vi "gyro-sweeper-module-V3.vi"(8 "fitter event pair":T4, 9 "async sweeper event pair":T4, 11 "this sweeper event pair":T4) -> ()   [LabVIEW 2018]
uses:
  cursor winow.ctl
  cursor window action.ctl
  KM_file -- read-write control.ctl
  filename-action.ctl
  file -- read-write control.ctl
  publisher action.ctl
  show-win- control.ctl
  server talkto message type.ctl
  filename-pattern.ctl
  server talkback message type.ctl
  server talk-to-back pair.ctl
panel:
  in  "sweeper panel":T1(tab)
  in  "sweep is ON":bool
  in  "win":T2={"cen (Hz)"=70746.20478327299, "win (Hz)"=2974.673840305428, "left (Hz)"=69258.86786312028, "right (Hz)"=72233.5417034257}
  out "Plot: circle sweep window":cluster{"Freq out (Hz)":dbl[], dbl[]}[](graph)
  in  "sweep! :r":bool
  in  "subtract bgnd!":bool
  in  "fit!":bool=TRUE
  in  "cursor window":T3={"left"=69258.86786312028, "right "=72233.5417034257, "center"=70746.20478327299, "window"=2974.673840305428, "cursors"=[0, 1, 2], "relative"=0, "absolute"=0, "fixed vertical offset"=0.0, "vertical offset"=0.0, "skew"=0.0, "default window frac"=0.1, "kind"=enum."symmetric", "skew.left"=0.5, "skew.right"=0.5, "Plot ref"=refnum, "wing order"=enum."forw"}
  in  "save data":enum32{"save/read"}(tab)
  in  "freqsweep name template":T5={"prefix"="RuCl3-rod", "group"="f"}
  in  "Save folder":path=path "/Users/Shared/Data"
  in  "freq sweep file name":string="f020_RuCl3-rod_042518.dat"
  in  "read from disk :l":bool
  in  "read file":path=path "/Users/arkady/Desktop/local_data/TaAs-quirk-Jan2018-losalamos/9w/f006_rucl3_012518.dat"
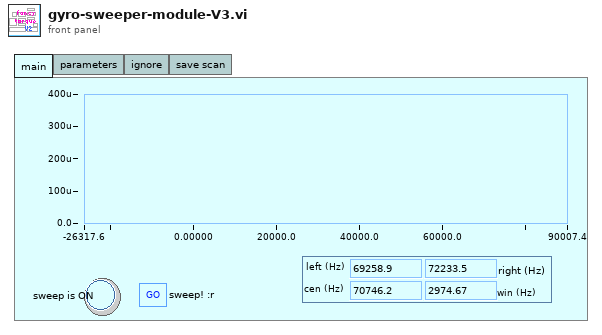
[diagram p1: front panel]
types:
  T1 = enum32{"main", "parameters", "ignore", "save scan"}
  T2 = typedef "show-win- control.ctl" = cluster{"cen (Hz)":dbl, "win (Hz)":dbl, "left (Hz)":dbl, "right (Hz)":dbl}
  T3 = typedef "cursor winow.ctl" = cluster{"left":dbl, "right ":dbl, "center":dbl, "window":dbl, "cursors":i32[], "relative":i32, "absolute":i32, "fixed vertical offset":dbl, "vertical offset":dbl, "skew":dbl, "default window frac":dbl, "kind":enum16{"symmetric", "skewed", "fancy"}, "skew.left":dbl, "skew.right":dbl, "Plot ref":refnum<vi>, "wing order":enum16{"forw", "back"}}
  T4 = typedef "server talk-to-back pair.ctl" = cluster{"talkback event":refnum<user-event>, "talkto event":refnum<user-event>}
  T5 = typedef "filename-pattern.ctl" = cluster{"prefix":string, "group":string}
  T6 = typedef "cursor window action.ctl" = enum16{"balance", "h. offset change", "cursor moves", "change center", "change window", "init", "check", "reset", "set y to middle", "idle", "-write all Y", "-write left.X", "-write center.X", "-write right.X", "-write all X", "-change center", "-change window", "-change skew", "-read cursor 2", "-read cursor 1", "-read cursor 0", "-read all cursors", "-reset", "-read plot scale", "-set y to middle", "-Q: center.Y is visible", "-Q: window is visible", "-parse center.Y", "-right left from center", "-left move", "-right move", "-set center.Y", "-empty", "-set cursors to default", "-check", "-write center.Y", "-copy cursor 1", "-copy cursor 0", "-copy cursor 2", "move right", "move left", "shrink", "broaden", "skew up", "skew down", "-write plot scale", "zoom X", "change cen&win", "zoom to all data", "color--red", "color--green", "color--yellow", "read", "zoom out", "zoom in", "slide right", "slide left", "set range aspect ratio to 1"}
  T7 = typedef "publisher action.ctl" = enum16{"set", "get", "init", "check"}
  T8 = typedef "file -- read-write control.ctl" = enum16{"read", "write all", "append one line"}
  T9 = typedef "filename-action.ctl" = enum16{"rewrite", "parse", "force pattern", "uniquenum"}
  T10 = typedef "KM_file -- read-write control.ctl" = enum16{"read", "write all", "append one line"}
  T11 = typedef "server talkto message type.ctl" = cluster{"message":enum16{"stop", "start", "update pars", "update request", "new", "launch", "exit", "get", "reset", "pause", "unpause"}}
  T12 = typedef "eventvkey.ctl" = enum16{"ASCII", "Enter", "Return", "Shift", "Ctrl", "Alt", "Cmd", "Opt", "Caps", "NumLock", "Clear", "Break", "Up", "Down", "Left", "Right", "Insert", "Delete", "Home", "End", "PageUp", "PageDown", "Escape", "Help", "Pause", "ScrollLock", "F1", "F2", "F3", "F4", "F5", "F6", "F7", "F8", "F9", "F10", "F11", "F12", "F13", "F14", "F15", "F16", "F17", "F18", "F19", "F20", "F21", "F22", "F23", "F24", "Play", "VolumeUp", "VolumeDown", "Mute", "Two Byte Char"}
  T13 = enum16{"stop", "start", "update pars", "update request", "new", "launch", "exit", "get", "reset", "pause", "unpause"}
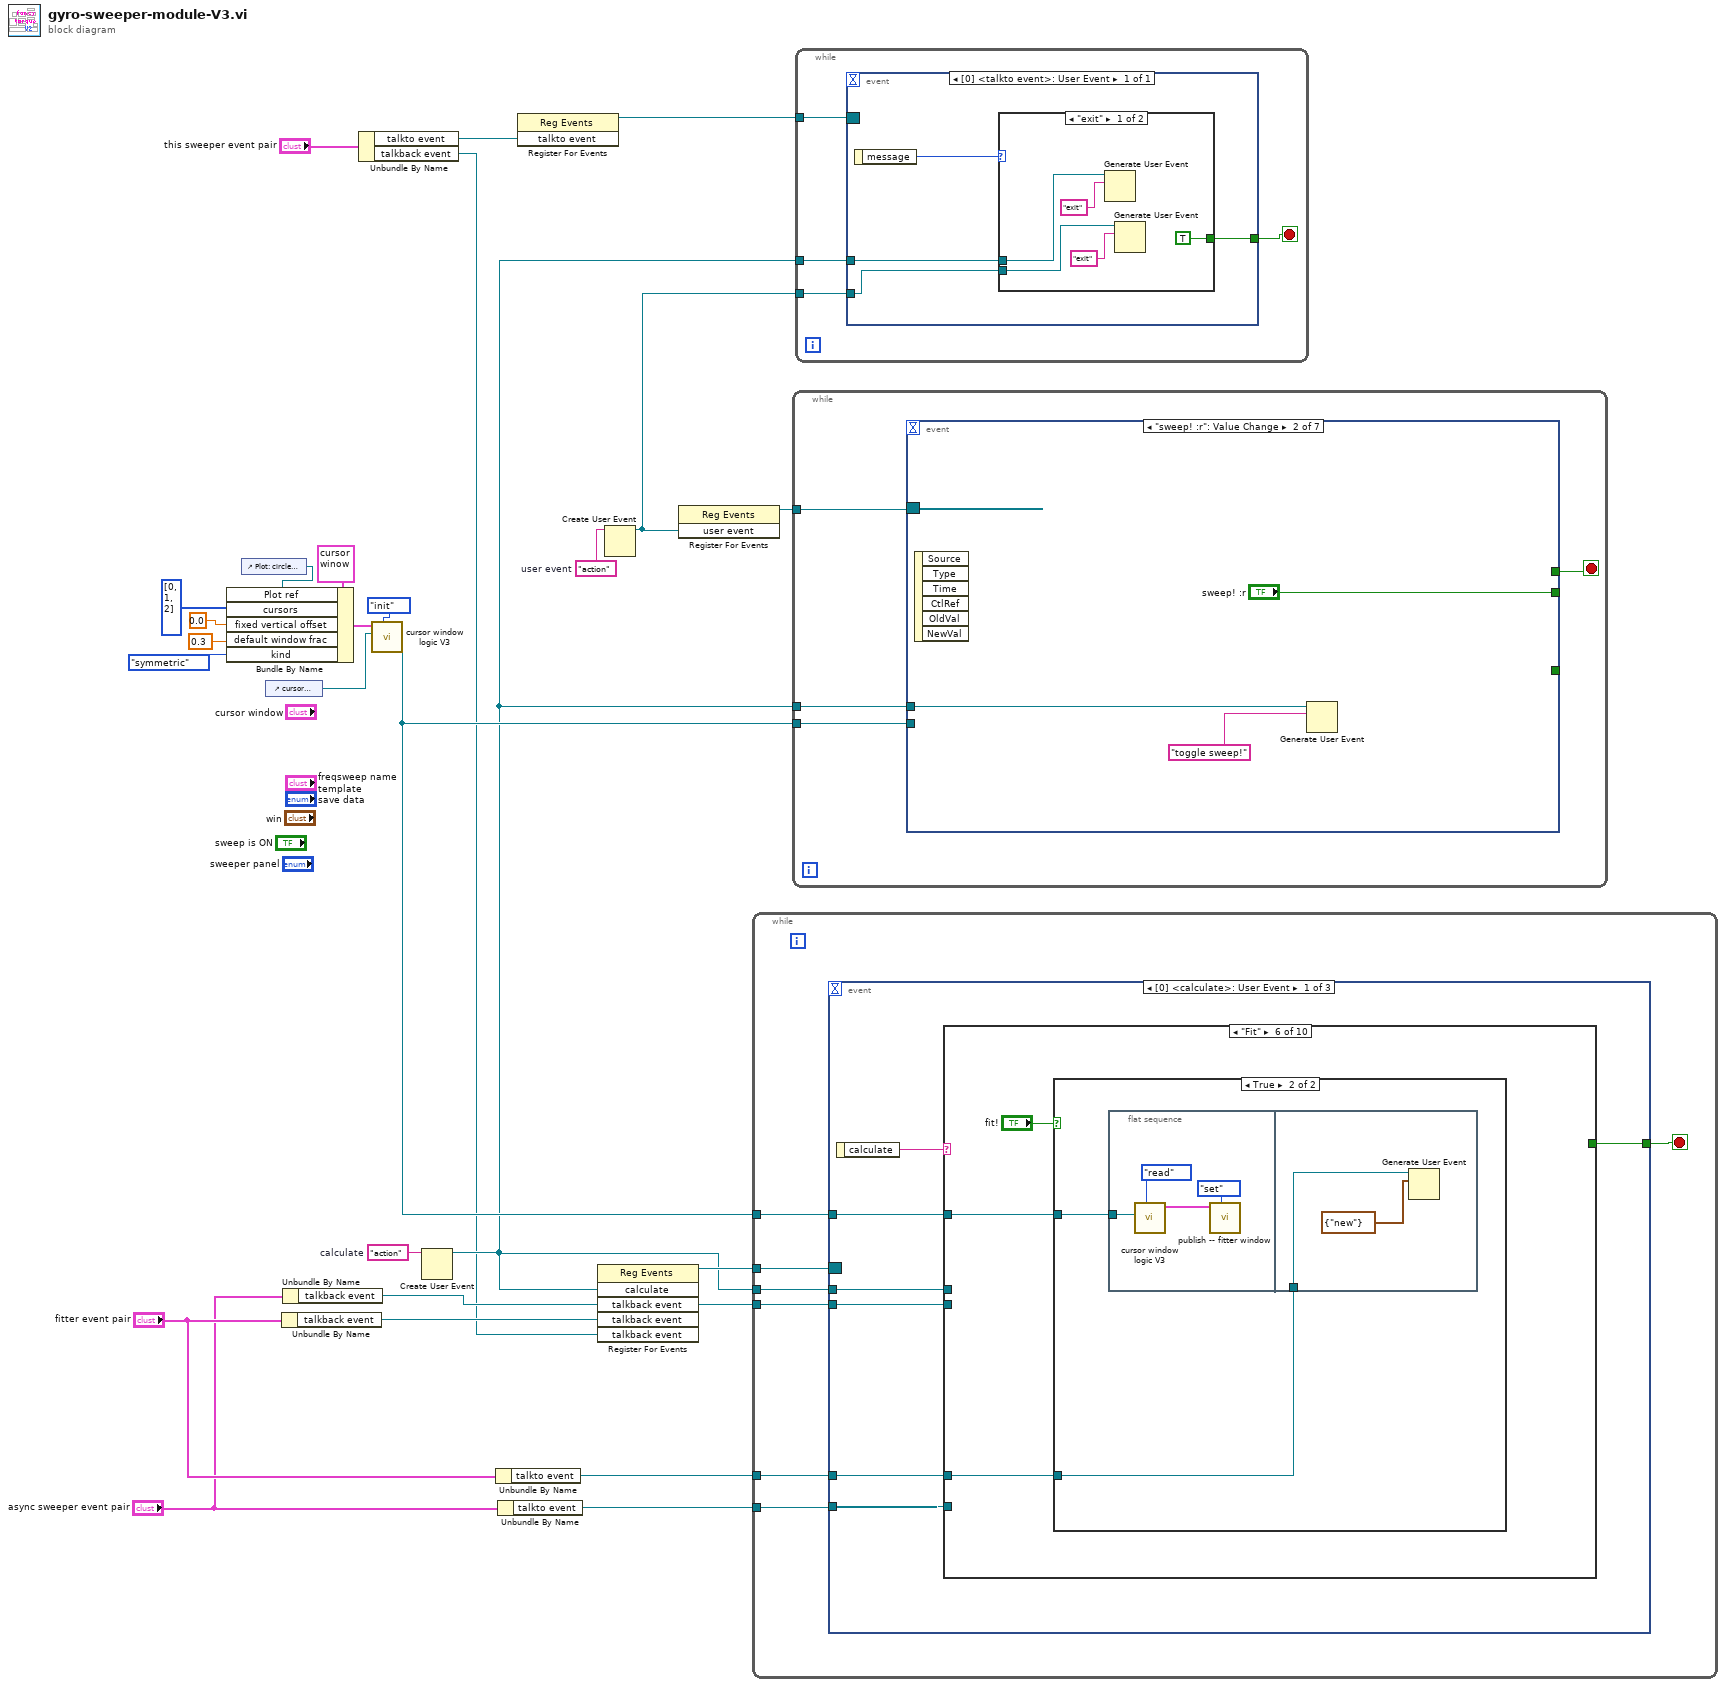
[diagram p0: block diagram]
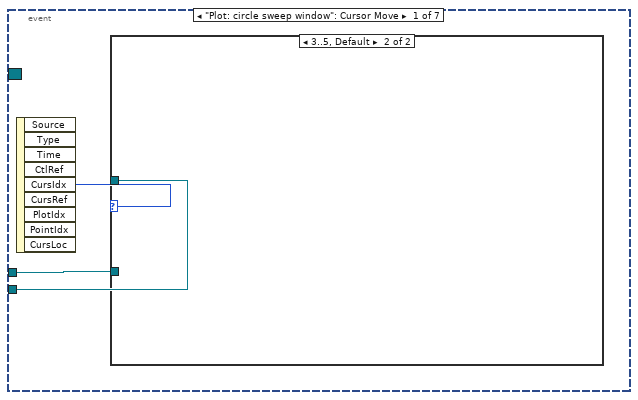
[diagram p3: hidden frame]
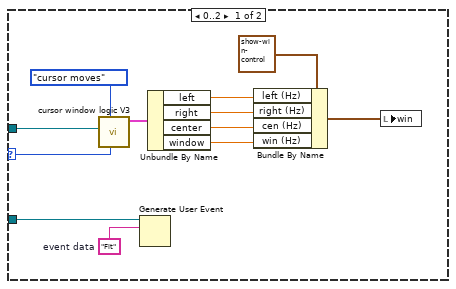
[diagram p4: hidden frame]
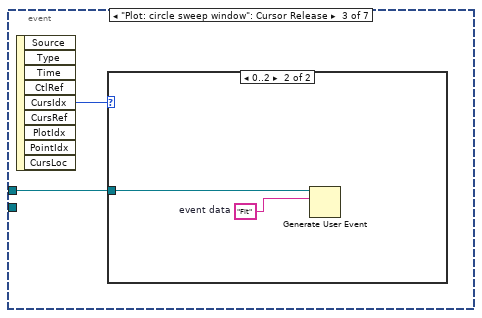
[diagram p5: hidden frame]
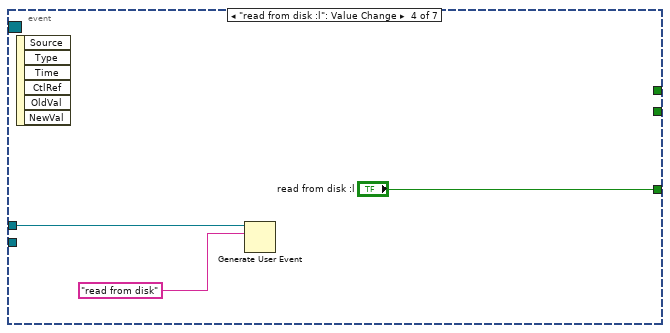
[diagram p7: hidden frame]
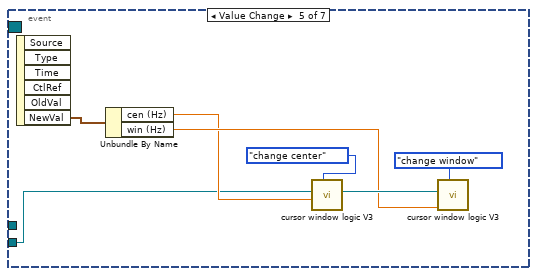
[diagram p8: hidden frame]
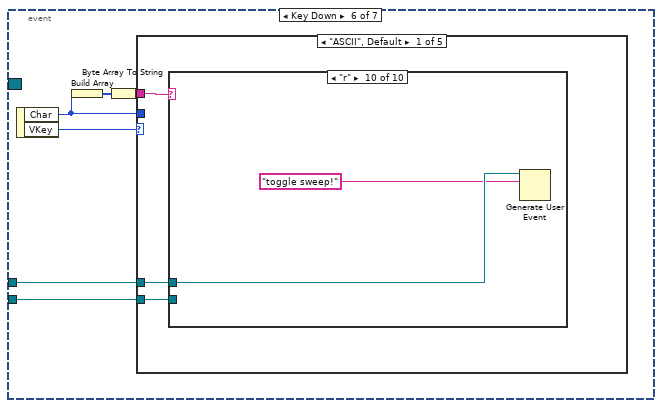
[diagram p9: hidden frame]
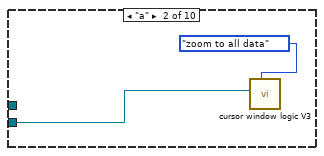
[diagram p11: hidden frame]
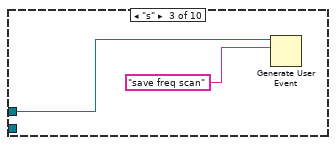
[diagram p12: hidden frame]
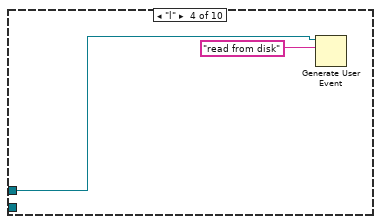
[diagram p13: hidden frame]
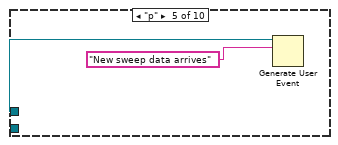
[diagram p14: hidden frame]
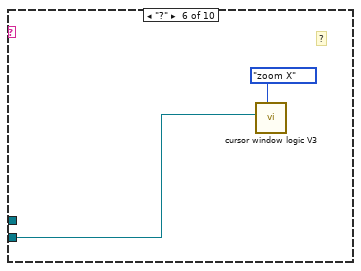
[diagram p15: hidden frame]
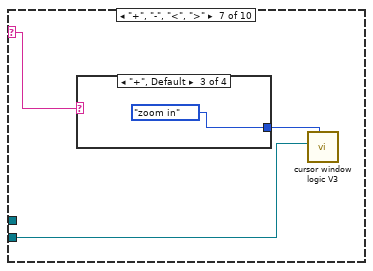
[diagram p16: hidden frame]
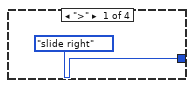
[diagram p17: hidden frame]
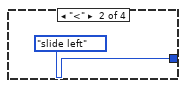
[diagram p18: hidden frame]
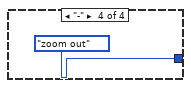
[diagram p19: hidden frame]
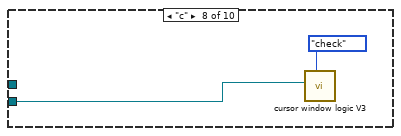
[diagram p20: hidden frame]
diagram:
  w23 = "action"  # user event
  w25 = "action"  # calculate
  n1 = control-ref of="Plot: circle sweep window"() -> (w14:refnum<vi>)
  n2 = Bundle By Name(cluster=T3 {"left"=0.0, "right "=0.0, "center"=0.0, "window"=0.0, "cursors"=[], "relative"=0, "absolute"=0, "fixed vertical offset"=0.0, "vertical offset"=0.0, "skew"=0.0, "default window frac"=0.0, "kind"=enum."symmetric", "skew.left"=0.0, "skew.right"=0.0, "Plot ref"=refnum, "wing order"=enum."forw"} ("cursor bracket: All, data window"), "Plot ref"=w14, "cursors"=i32[] [0, 1, 2], "fixed vertical offset"=0.0, "default window frac"=0.3 ("fixed vertical offset"), "kind"=enum16{"symmetric", "skewed", "fancy"}."symmetric") -> (w18:T3)
  n3 = control-ref of="cursor window"() -> (w13:refnum<vi>)
  n4 = Unbundle By Name("fitter event pair") -> ("talkback event"=w9:refnum<user-event>)
  n5 = Unbundle By Name("async sweeper event pair") -> ("talkback event"=w7:refnum<user-event>)
  n6 = Unbundle By Name("this sweeper event pair") -> ("talkto event"=w4:refnum<user-event>, "talkback event"=w1:refnum<user-event>)
  n7 = call "cursor window logic V3.vi"("cursor window action"=cursor_window_action."init", "cursor window in"=w13, "cursor window init"=w18) -> ("cursor window out"=w16:refnum<vi>)  [unwired: 7 in, 1 out]
  n8 = Create User Event(user event datatype=w25) -> (user event=w2:refnum<user-event>)  [unwired: 1 in, 1 out]
  n9 = Unbundle By Name("fitter event pair") -> ("talkto event"=w11:refnum<user-event>)
  n10 = Unbundle By Name("async sweeper event pair") -> ("talkto event"=w12:refnum<user-event>)
  n11 = register-events(w4) -> (reference out=w6:refnum<event-registration>)  [unwired: 2 in, 1 out]
  n12 = register-events(w2, w7, w9, w1) -> (reference out=w26:refnum<event-registration>)  [unwired: 2 in, 1 out]
  n13 = Create User Event(user event datatype=w23) -> (user event=w3:refnum<user-event>)  [unwired: 1 in, 1 out]
  n14 = register-events(w3) -> (reference out=w24:refnum<event-registration>)  [unwired: 2 in, 1 out]
  n15 = while {
    tunnel: w26 -> [w33]
    tunnel: w2 -> [w32]
    tunnel: w16 -> [w31]
    tunnel: w12 -> [w30]
    tunnel: w7 -> [w29]
    tunnel: w11 -> [w28]
    stop <- w27 stop-if-true
    n16 = event shown="[0] <calculate>: User Event" {
      selector: w33 -> [_ _ _]
      dyn-events: _ -> [_ _ _]
      timeout: _ -> [_ _ _]
      tunnel: w32 -> [w39 w132 _]
      tunnel: w31 -> [w38 _ _]
      tunnel: w30 -> [w37 _ _]
      tunnel: w29 -> [w36 _ _]
      tunnel: w28 -> [w35 _ _]
      tunnel: [w34 _ _] -> w27
      event User Event {
        n17 = event-data() -> ("calculate"=w40:string)  [unwired: 1 in]
        n18 = case shown="\"Fit\"" w40 {
          tunnel: w39 -> [w49 w72 _ w77 _ _ _ _ _ _]
          tunnel: w38 -> [_ _ _ _ _ w109 _ _ _ _]
          tunnel: w37 -> [_ _ _ _ _ _ w122 w127 w131 _]
          tunnel: w36 -> [_ _ _ _ _ _ _ _ _ _]
          tunnel: w35 -> [_ _ _ _ _ w107 _ _ _ _]
          tunnel: [_ _ TRUE _ _ _ _ _ _ _] -> w34
          frame "New sweep data arrives" {
            n19 = call "MFLI -- publish -- freq scan.vi"("publisher action"=publisher_action."get") -> ("Voltage out (V)"=w46:cdb[], "Freq out (Hz)"=w48:dbl[])  [unwired: 9 in]
            n20 = Generate User Event(user event=w49, event data cluster="Fit" ("event data")) -> ()  [unwired: 2 in, 2 out]
            n21 = case shown="False" "subtract bgnd!" {
              tunnel: w48 -> [w61 w69]
              tunnel: [w55 w69] -> w47
              tunnel: w46 -> [w57 w68]
              tunnel: [w62 w68] -> w45
              frame True {
                w54 = 10 ("length")
                n22 = Delete From Array(array=w61, length=w54, index=0) -> (array with subset deleted=w60:dbl[])  [unwired: 1 out]
                n23 = Delete From Array(array=w57, length=w54, index=0) -> (array with subset deleted=w56:cdb[])  [unwired: 1 out]
                n24 = call "linear interp iiii- complex - z-omega.vi"("z"=w56, "omega"=w60) -> ("z out"=w63:cdb[], "omega out"=w55:dbl[], "intercept"=w65:cdb, "slope"=w66:cdb)  [unwired: 5 in, 5 out]
                n25 = Multiply(x=w55, y=w66) -> (x*y=w67:cdb[])
                n26 = Add(x=w67, y=w65) -> (x+y=w64:cdb[])
                n27 = Subtract(x=w63, y=w64) -> (x-y=w62:cdb[])
              }
              frame False {
              }
            }
            n28 = Complex To Re/Im(x + iy=w45) -> (x=w52:dbl[], y=w51:dbl[])
            n29 = Bundle("Freq out (Hz)"=w47, w52) -> (w53:cluster{"Freq out (Hz)":dbl[], dbl[]})  [unwired: 1 in]
            n30 = Bundle("Freq out (Hz)"=w47, w51) -> (w50:cluster{"Freq out (Hz)":dbl[], dbl[]})  [unwired: 1 in]
            n31 = Build Array(w53, w50) -> (→"Plot: circle sweep window":cluster{"Freq out (Hz)":dbl[], dbl[]}[])
          }
          frame "toggle sweep!" {
            n32 = local read "sweep is ON"() -> (w71:bool)
            n33 = case shown="False" w71 {
              tunnel: ["start sweep!" ("event data") "stop sweep!" ("event data")] -> w70
              frame False {
              }
              frame True {
              }
            }
            n34 = Generate User Event(user event=w72, event data cluster=w70) -> ()  [unwired: 2 in, 2 out]
          }
          frame "exit" {
            n35 = local write "sweep is ON"(FALSE ("sweep ON")) -> ()
          }
          frame "read from disk" {
            n36 = call "file - read-write - list of lines.vi"("read/write control"=file_--_read-write_control."read", "file path"="read file") -> ("list of lines OUT"=w81:string[])  [unwired: 8 in, 1 out]
            n37 = for {
              tunnel: w81 -> [w91] mode=indexing
              tunnel: [w86] -> w82 mode=indexing
              tunnel: [w85] -> w83 mode=indexing
              w87 = 0.0
              n38 = Scan From String(format string="%f%f%f", input string=w91, default 1=w87, default 2=w87, default 3=w87) -> (output 1=w85:dbl, output 2=w89:dbl, output 3=w88:dbl)  [unwired: 2 in, 3 out]
              n39 = Re/Im To Complex(1:w88, 2:w89) -> (0:w86:cdb)
            }
            n40 = flat-sequence {
              tunnel: w77 -> [w95]
              tunnel: [w95] -> w84
              tunnel: w82 -> [w93]
              tunnel: w83 -> [w92]
              tunnel: w84 -> [w97]
              tunnel: "New sweep data arrives" ("event data") -> [w96]
              frame #0 {
                n41 = call "MFLI -- publish -- freq scan.vi"("publisher action"=publisher_action."set", "Voltage IN (V)"=w93, "Freq IN (Hz)"=w92) -> ()  [unwired: 7 in, 2 out]
              }
              frame #1 {
                n42 = Generate User Event(user event=w97, event data cluster=w96) -> ()  [unwired: 2 in, 2 out]
              }
            }
          }
          frame "save freq scan" {
            n43 = local read "freqsweep name template"() -> (w103:T5)
            n44 = call "MFLI -- publish -- freq scan.vi"("publisher action"=publisher_action."get") -> ("Voltage out (V)"=w99:cdb[], "Freq out (Hz)"=w100:dbl[])  [unwired: 9 in]
            n45 = call "filename-manage.vi"("filename pattern"=w103, "filename-action"=filename-action."uniquenum", "folder"="Save folder", "file name"="freq sweep file name") -> ("filename OUT"=w102:string)  [unwired: 7 in]
            n46 = call "KM_appendline -- freq sweep.vi"("freq"=w100, "Vout(V)"=w99, "Save frequency scan"="Save folder", "read/write control"=KM_file_--_read-write_control."append one line", "name or relative path"=w102) -> ()  [unwired: 15 in]
            n47 = local write "freq sweep file name"(w102) -> ()
          }
          frame "Fit" {
            n48 = case shown="True" "fit!" {
              tunnel: w109 -> [_ w111]
              tunnel: w107 -> [_ w110]
              frame False {
              }
              frame True {
                n49 = flat-sequence {
                  tunnel: w111 -> [w114]
                  tunnel: w110 -> [w116]
                  frame #0 {
                    n50 = call "cursor window logic V3.vi"("cursor window action"=cursor_window_action."read", "cursor window in"=w114) -> ("cursor window out"=w113:T3)  [unwired: 8 in, 1 out]
                    n51 = call "publish -- fitter window.vi"("publisher action"=publisher_action."set", "win IN"=w113) -> ()  [unwired: 9 in, 1 out]
                  }
                  frame #1 {
                    n52 = Generate User Event(user event=w116, event data cluster=T11 {"message"=enum."new"} ("event data")) -> ()  [unwired: 2 in, 2 out]
                  }
                }
              }
            }
          }
          frame "start sweep!" {
            n53 = local read "win"() -> (w119:T2)
            n54 = call "publish -- sweeper window.vi"("publisher action"=publisher_action."set", "win IN"=w119) -> ()  [unwired: 9 in, 1 out]
            n55 = local write "sweep is ON"(TRUE ("sweep ON")) -> ()
            n56 = Generate User Event(user event=w122, event data cluster=T11 {"message"=enum."update request"} ("event data")) -> (user event out=w121:refnum<user-event>)  [unwired: 2 in, 1 out]
            n57 = Generate User Event(user event=w121, event data cluster=T11 {"message"=enum."start"} ("event data")) -> ()  [unwired: 2 in, 2 out]
          }
          frame "stop sweep!" {
            n58 = Generate User Event(user event=w127, event data cluster=T11 {"message"=enum."stop"} ("event data")) -> ()  [unwired: 2 in, 2 out]
            n59 = local write "sweep is ON"(FALSE ("sweep ON")) -> ()
          }
          frame "update win" {
            n60 = local read "win"() -> (w128:T2)
            n61 = call "publish -- sweeper window.vi"("publisher action"=publisher_action."set", "win IN"=w128) -> ()  [unwired: 9 in, 1 out]
            n62 = Generate User Event(user event=w131, event data cluster=T11 {"message"=enum."update request"} ("event data")) -> ()  [unwired: 2 in, 2 out]
          }
          frame "Void", Default {
          }
        }
      }
      event User Event {
        n63 = event-data() -> ("message"=w133:enum16{"new", "void"})  [unwired: 1 in, 4 out]
        n64 = case shown="\"new\", Default" w133 {
          tunnel: w132 -> [w134]
          frame "new", Default {
            n65 = Generate User Event(user event=w134, event data cluster="New sweep data arrives" ("event data")) -> ()  [unwired: 2 in, 2 out]
          }
        }
      }
      event User Event {
        n66 = event-data() -> ()  [unwired: 1 in, 1 out]
      }
    }
  }
  n67 = while {
    tunnel: w24 -> [w139]
    tunnel: w2 -> [w138]
    tunnel: w16 -> [w137]
    stop <- w136 stop-if-true
    n68 = event shown="[1] \"sweep! :r\": Value Change" {
      selector: w139 -> [_ _ _ _ _ _ _]
      dyn-events: _ -> [_ _ _ _ _ _ _]
      timeout: _ -> [_ _ _ _ _ _ _]
      tunnel: w138 -> [w140 w157 w159 w164 _ w176 _]
      tunnel: w137 -> [w142 _ _ _ w165 w172 _]
      tunnel: [_ "sweep! :r" _ _ _ _ _] -> _
      tunnel: [_ _ _ "read from disk :l" _ _ _] -> _
      tunnel: [_ _ _ _ _ _ w220] -> w136
      event "Plot: circle sweep window": Cursor Move {
        n69 = event-data() -> ("CursIdx"=w141:i32)  [unwired: 1 in, 8 out]
        n70 = case shown="3..5, Default" w141 {
          selector: w141 -> [w152 _]
          tunnel: w142 -> [w154 _]
          tunnel: w140 -> [w150 _]
          frame 0..2 {
            w149 = "Fit"  # event data
            n71 = call "cursor window logic V3.vi"("CursIdx"=w152, "cursor window action"=cursor_window_action."cursor moves", "cursor window in"=w154) -> ("cursor window out"=w151:T3)  [unwired: 7 in, 1 out]
            n72 = Generate User Event(user event=w150, event data cluster=w149) -> ()  [unwired: 2 in, 2 out]
            n73 = Unbundle By Name(w151) -> ("left"=w146:dbl, "right"=w145:dbl, "center"=w144:dbl, "window"=w143:dbl)
            n74 = Bundle By Name(cluster=T2 {"cen (Hz)"=-0.35260838541595674, "win (Hz)"=17.234446484426172, "left (Hz)"=-8.969831627629043, "right (Hz)"=8.26461485679713} ("win"), "left (Hz)"=w146, "right (Hz)"=w145, "cen (Hz)"=w144, "win (Hz)"=w143) -> (w147:T2)
            n75 = local write "win"(w147) -> ()
          }
          frame 3..5, Default {
          }
        }
      }
      event "sweep! :r": Value Change {
        n76 = event-data() -> ()  [unwired: 1 in, 6 out]
        n77 = Generate User Event(user event=w157, event data cluster="toggle sweep!" ("event data")) -> ()  [unwired: 2 in, 2 out]
      }
      event "Plot: circle sweep window": Cursor Release {
        n78 = event-data() -> ("CursIdx"=w158:i32)  [unwired: 1 in, 8 out]
        n79 = case shown="0..2" w158 {
          tunnel: w159 -> [_ w160]
          frame 3, Default {
          }
          frame 0..2 {
            w161 = "Fit"  # event data
            n80 = Generate User Event(user event=w160, event data cluster=w161) -> ()  [unwired: 2 in, 2 out]
          }
        }
      }
      event "read from disk :l": Value Change {
        n81 = event-data() -> ()  [unwired: 1 in, 6 out]
        n82 = Generate User Event(user event=w164, event data cluster="read from disk" ("event data")) -> ()  [unwired: 2 in, 2 out]
      }
      event Value Change {
        n83 = event-data() -> ("NewVal"=w168:T2)  [unwired: 1 in, 5 out]
        n84 = Unbundle By Name(w168) -> ("cen (Hz)"=w166:dbl, "win (Hz)"=w167:dbl)
        n85 = call "cursor window logic V3.vi"("cursor window action"=cursor_window_action."change center", "center"=w166, "cursor window in"=w165) -> ("cursor window out"=w169:refnum<vi>)  [unwired: 7 in, 1 out]
        n86 = call "cursor window logic V3.vi"("cursor window action"=cursor_window_action."change window", "window"=w167, "cursor window in"=w169) -> ()  [unwired: 7 in, 2 out]
      }
      event Key Down {
        n87 = event-data() -> ("Char"=w174:i16, "VKey"=w177:T12)  [unwired: 1 in]
        n88 = Build Array(w174) -> (w175:i16[])
        n89 = Byte Array To String(unsigned byte array=w175) -> (string=w173:string)
        n90 = case shown="\"ASCII\", Default" w177 {
          selector: w177 -> [_ _ _ _ w215]
          tunnel: w174 -> [_ _ _ _ _]
          tunnel: w176 -> [w180 _ _ _ w214]
          tunnel: w173 -> [w179 _ _ _ _]
          tunnel: w172 -> [w178 _ _ _ w211]
          frame "ASCII", Default {
            n91 = case shown="\"r\"" w179 {
              selector: w179 -> [_ _ _ _ _ _ w192 _ _ _]
              tunnel: w180 -> [_ _ w183 w185 w187 _ _ _ _ w201]
              tunnel: w178 -> [_ w181 _ _ _ w189 w193 w198 _ _]
              frame "0", Default {
              }
              frame "a" {
                n92 = call "cursor window logic V3.vi"("cursor window action"=cursor_window_action."zoom to all data", "cursor window in"=w181) -> ()  [unwired: 8 in, 2 out]
              }
              frame "s" {
                n93 = Generate User Event(user event=w183, event data cluster="save freq scan" ("event data")) -> ()  [unwired: 2 in, 2 out]
              }
              frame "l" {
                n94 = Generate User Event(user event=w185, event data cluster="read from disk" ("event data")) -> ()  [unwired: 2 in, 2 out]
              }
              frame "p" {
                n95 = Generate User Event(user event=w187, event data cluster="New sweep data arrives" ("event data")) -> ()  [unwired: 2 in, 2 out]
              }
              frame "?" {
                # "?"
                n96 = call "cursor window logic V3.vi"("cursor window action"=cursor_window_action."zoom X", "cursor window in"=w189) -> ()  [unwired: 8 in, 2 out]
              }
              frame "+", "-", "<", ">" {
                n97 = case shown="\"+\", Default" w192 {
                  tunnel: [cursor_window_action."slide right" ("cursor window action") cursor_window_action."slide left" ("cursor window action") cursor_window_action."zoom in" ("cursor window action") cursor_window_action."zoom out" ("cursor window action")] -> w191
                  frame ">" {
                  }
                  frame "<" {
                  }
                  frame "+", Default {
                  }
                  frame "-" {
                  }
                }
                n98 = call "cursor window logic V3.vi"("cursor window action"=w191, "cursor window in"=w193) -> ()  [unwired: 8 in, 2 out]
              }
              frame "c" {
                n99 = call "cursor window logic V3.vi"("cursor window action"=cursor_window_action."check", "cursor window in"=w198) -> ()  [unwired: 8 in, 2 out]
              }
              frame "t" {
              }
              frame "r" {
                n100 = Generate User Event(user event=w201, event data cluster="toggle sweep!" ("event data")) -> ()  [unwired: 2 in, 2 out]
              }
            }
          }
          frame "Escape" {
          }
          frame "PageUp" {
          }
          frame "PageDown" {
          }
          frame "Up".."Right" {
            w202 = "update win"  # event data
            w204 = "Fit"  # event data
            n101 = case shown="\"Left\"" w215 {
              tunnel: [cursor_window_action."move right" ("cursor window action") cursor_window_action."move left" ("cursor window action") cursor_window_action."broaden" ("cursor window action") cursor_window_action."shrink" ("cursor window action")] -> w213
              frame "Right", Default {
              }
              frame "Left" {
              }
              frame "Up" {
              }
              frame "Down" {
              }
            }
            n102 = call "cursor window logic V3.vi"("cursor window action"=w213, "cursor window in"=w211) -> ("cursor window out"=w212:T3)  [unwired: 8 in, 1 out]
            n103 = Unbundle By Name(w212) -> ("left"=w208:dbl, "right"=w207:dbl, "center"=w206:dbl, "window"=w205:dbl)
            n104 = Generate User Event(user event=w214, event data cluster=w204) -> (user event out=w203:refnum<user-event>)  [unwired: 2 in, 1 out]
            n105 = Bundle By Name(cluster=T2 {"cen (Hz)"=-0.35260838541595674, "win (Hz)"=17.234446484426172, "left (Hz)"=-8.969831627629043, "right (Hz)"=8.26461485679713} ("win"), "left (Hz)"=w208, "right (Hz)"=w207, "cen (Hz)"=w206, "win (Hz)"=w205) -> (w210:T2)
            n106 = Generate User Event(user event=w203, event data cluster=w202) -> ()  [unwired: 2 in, 2 out]
            n107 = local write "win"(w210) -> ()
          }
        }
      }
      event User Event {
        n108 = event-data() -> ("user event"=w221:string)  [unwired: 1 in, 4 out]
        n109 = case shown="\"exit\"" w221 {
          tunnel: [_ TRUE] -> w220
          frame "False", Default {
          }
          frame "exit" {
          }
        }
      }
    }
  }
  n110 = while {
    tunnel: w6 -> [w226]
    tunnel: w2 -> [w224]
    tunnel: w3 -> [w223]
    stop <- w225 stop-if-true
    n111 = event shown="[0] <talkto event>: User Event" {
      selector: w226 -> [_]
      dyn-events: _ -> [_]
      timeout: _ -> [_]
      tunnel: [w229] -> w225
      tunnel: w224 -> [w228]
      tunnel: w223 -> [w227]
      event User Event {
        n112 = event-data() -> ("message"=w230:T13)  [unwired: 1 in]
        n113 = case shown="\"exit\"" w230 {
          tunnel: [TRUE _] -> w229
          tunnel: w228 -> [w234 _]
          tunnel: w227 -> [w231 _]
          frame "exit" {
            n114 = Generate User Event(user event=w234, event data cluster="exit" ("event data")) -> ()  [unwired: 2 in, 2 out]
            n115 = Generate User Event(user event=w231, event data cluster="exit" ("event data")) -> ()  [unwired: 2 in, 2 out]
          }
          frame "start", Default {
          }
        }
      }
    }
  }
